vi "LHF.DB.Mongo.Bson.MultiDArray.vi"(8 "error in (no error)":errorcluster, 10 "Array Dimensions":i32[](array[numeric]), 11 "Variant Data":T1[](array[typedef])) -> (0 "error out":errorcluster, 2 "BsonArray":refnum<k24>, 3 "Remaining Variant Data":T1[](array[typedef]))   [LabVIEW 2013, in "LHF.DB.Mongo.lvclass"]
uses:
  LHF.DB.Mongo.lvclass
  Typedef/LHF.DB.Mongo.Typedef.VariantData.ctl
  <vilib>/Utility/VariantDataType/Type.ctl
  C:/Users/schim/Desktop/Projetos/LabVIEW-MongoDB/src/Driver/MongoDB.Bson.dll
  Driver/MongoDB.Bson.dll
  <vilib>/Utility/VariantDataType/VariantType.lvlib
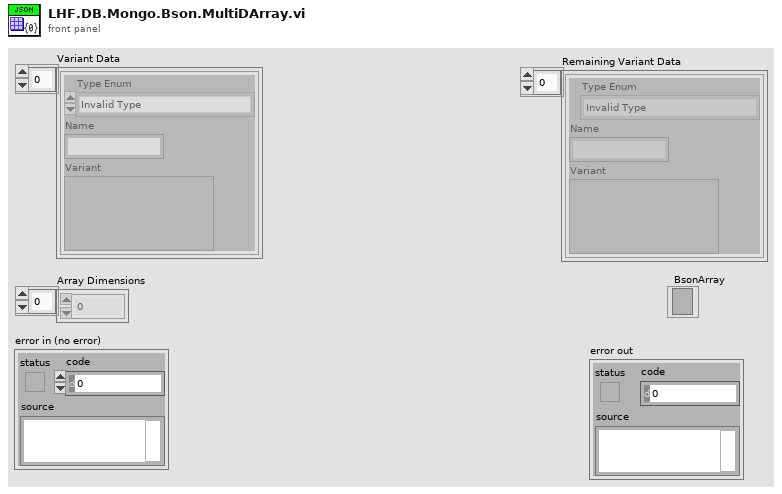
[diagram p1: front panel]
types:
  T1 = typedef "LHF.DB.Mongo.lvclass/LHF.DB.Mongo.Typedef.VariantData.ctl" = cluster{"Type Enum":T2, "Name":string, "Variant":variant}
  T2 = typedef "VariantType.lvlib/Type.ctl" = enum8{"Invalid Type", "Void", "I8", "I16", "I32", "I64", "U8", "U16", "U32", "U64", "Single Float", "Double Float", "Extended Float", "Single Complex", "Double Complex", "Extended Complex", "Enum U8", "Enum U16", "Enum U32", "Enum U64", "Single Float With Unit", "Double Float With Unit", "Extended Float With Unit", "Single Complex with Unit", "Double Complex with Unit", "Extended Complex with Unit", "Boolean", "String", "Path", "Picture", "Tag", "Array", "Cluster", "Variant", "LV Variant", "Waveform", "Timestamp", "Digital Waveform", "Digital Data", "ExpressData", "Refnum", "External Data", "VI", "Poly VI", "LabVIEW Class Instance", "Fixed Point"}
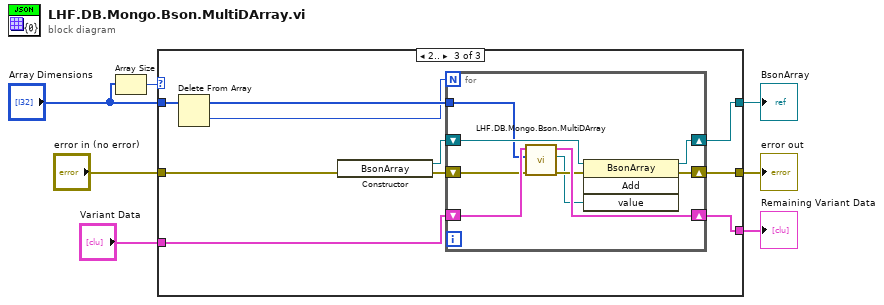
[diagram p0: block diagram]
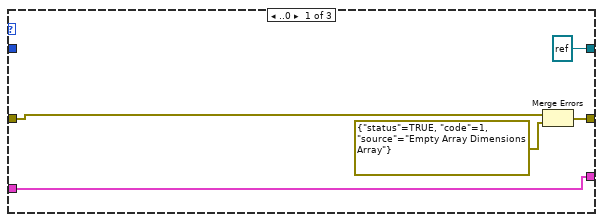
[diagram p2: hidden frame]
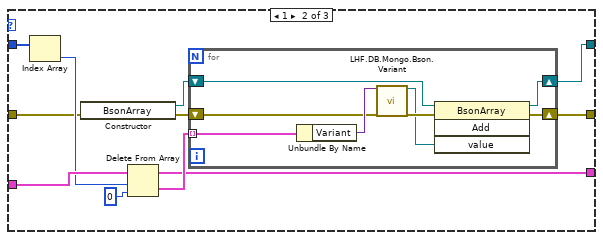
[diagram p3: hidden frame]
diagram:
  n1 = Array Size(array="Array Dimensions") -> (size(s)=w4:i32)
  n2 = case shown="2.." w4 {
    tunnel: "Variant Data" -> [w11 w22 w33]
    tunnel: "error in (no error)" -> [w12 w15 w38]
    tunnel: [w10 w13 w37] -> w5
    tunnel: [refnum<k24> refnum ("new reference") w16 w34] -> w1
    tunnel: "Array Dimensions" -> [_ w23 w41]
    tunnel: [w11 w19 w32] -> w2
    frame ..0 {
      n3 = Merge Errors(w12, errorcluster {"status"=TRUE, "code"=1, "source"="Empty Array Dimensions Array"} ("error in")) -> (w10:errorcluster)
    }
    frame 1 {
      n4 = Index Array(array=w23) -> (element=w21:i32)  [unwired: 1 in]
      n5 = constructor class="BsonArray"(error in=w15) -> (reference out=w17:refnum<k24>, error out=w14:errorcluster)  [unwired: 2 in, 1 out]
      n6 = Delete From Array(array=w22, length=w21, index=0) -> (deleted portion=w20:T1[], array with subset deleted=w19:T1[])
      n7 = for {
        tunnel: w20 -> [w31] mode=indexing
        shift-right: [w24] -> w13
        shift-left: w14 -> [w25]
        shift-right: [w26] -> w16
        shift-left: w17 -> [w28]
        n8 = Unbundle By Name(w31) -> ("Variant"=w30:variant)
        n9 = call "LHF.DB.Mongo.Bson.Variant.vi"("Variant"=w30, "error IO"=w25) -> ("BsonValue"=w27:refnum<k24>, "error IO 2"=w29:errorcluster)  [unwired: 16 in]
        n10 = invoke class="BsonArray" method="Add"(reference=w28, error in=w29, "value"=w27) -> (reference out=w26:refnum<k24>, error out=w24:errorcluster)  [unwired: 1 in, 2 out]
      }
    }
    frame 2.. {
      n11 = Delete From Array(array=w41) -> (deleted portion=w35:i32, array with subset deleted=w36:i32[])  [unwired: 2 in]
      n12 = constructor class="BsonArray"(error in=w38) -> (reference out=w40:refnum<k24>, error out=w39:errorcluster)  [unwired: 2 in, 1 out]
      n13 = for {
        N: w35 -> [_]
        shift-right: [w43] -> w37
        shift-left: w39 -> [w44]
        shift-right: [w48] -> w32
        shift-left: w33 -> [w47]
        shift-right: [w50] -> w34
        shift-left: w40 -> [w49]
        tunnel: w36 -> [w46]
        n14 = call "LHF.DB.Mongo.Bson.MultiDArray.vi"("error in (no error)"=w44, "Array Dimensions"=w46, "Variant Data"=w47) -> ("error out"=w45:errorcluster, "BsonArray"=w42:refnum<k24>, "Remaining Variant Data"=w48:T1[])  [unwired: 6 in]
        n15 = invoke class="BsonArray" method="Add"(reference=w49, error in=w45, "value"=w42) -> (reference out=w50:refnum<k24>, error out=w43:errorcluster)  [unwired: 1 in, 2 out]
      }
    }
  }
  "error out" <- w5
  "BsonArray" <- w1
  "Remaining Variant Data" <- w2
